vi "Folder Setting.vi"(8 "error in":errorcluster, 10 "Folder containing database files":path=path "C:/MHWirth/Data Logging Application/Logs/Database", 11 "Folder for saving log files":path=path "C:/MHWirth/Data Logging Application/Logs/Database") -> (0 "error out":errorcluster, 2 "database folder":path, 3 "TDMS folder":path)   [LabVIEW 2014]
doc: "<B>Copyrights</B>: (c) MHWirth 2015. All rights reserved.\n\nThis subVI updates the path for folders \"to save TDMS file\" and \"to contain the database\"."
panel:
  in  "update":bool
  # "Settings - Folder"
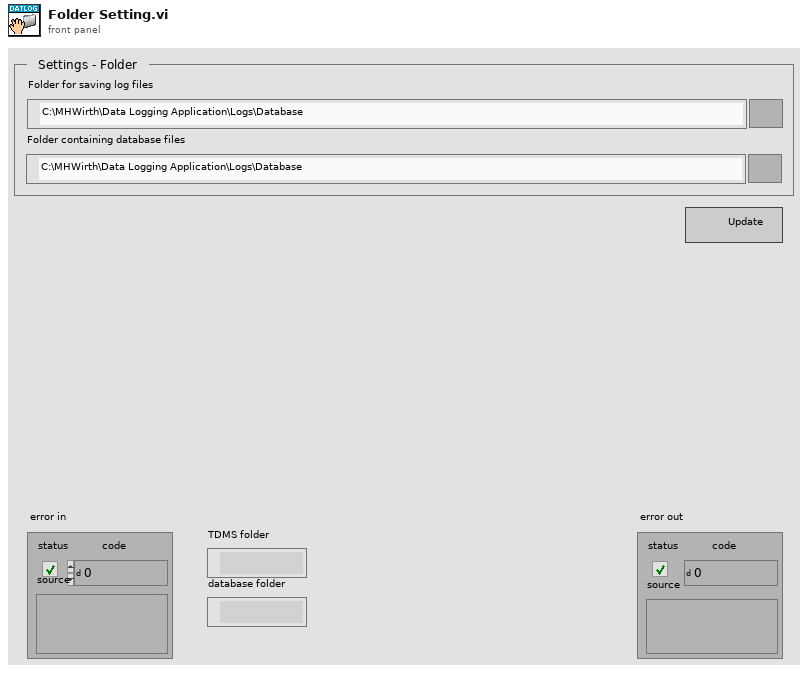
[diagram p1: front panel]
types:
  T1 = typedef "eventvkey.ctl" = enum16{"ASCII", "Enter", "Return", "Shift", "Ctrl", "Alt", "Cmd", "Opt", "Caps", "NumLock", "Clear", "Break", "Up", "Down", "Left", "Right", "Insert", "Delete", "Home", "End", "PageUp", "PageDown", "Escape", "Help", "Pause", "ScrollLock", "F1", "F2", "F3", "F4", "F5", "F6", "F7", "F8", "F9", "F10", "F11", "F12", "F13", "F14", "F15", "F16", "F17", "F18", "F19", "F20", "F21", "F22", "F23", "F24", "Play", "VolumeUp", "VolumeDown", "Mute", "Two Byte Char"}
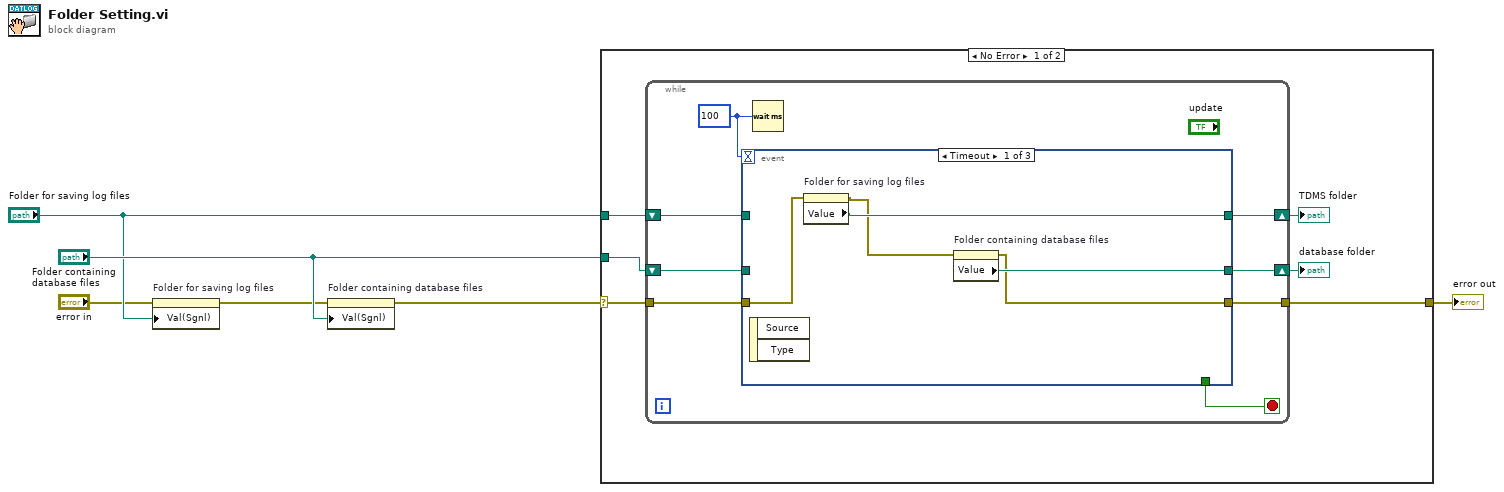
[diagram p0: block diagram]
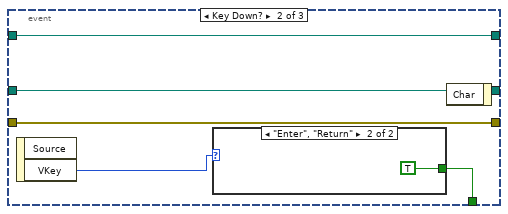
[diagram p2: hidden frame]
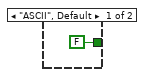
[diagram p3: hidden frame]
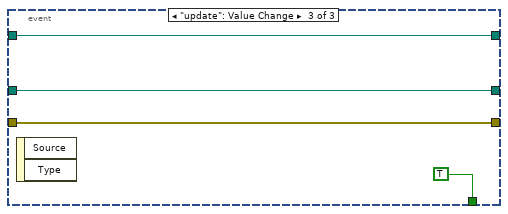
[diagram p4: hidden frame]
diagram:
  n1 = property on="Folder for saving log files" class="Path"(error in="error in", "Val(Sgnl)"="Folder for saving log files") -> (error out=w1:errorcluster)  [unwired: 1 in, 1 out]
  n2 = property on="Folder containing database files" class="Path"(error in=w1, "Val(Sgnl)"="Folder containing database files") -> (error out=w5:errorcluster)  [unwired: 1 in, 1 out]
  n3 = case shown="No Error" w5 {
    selector: w5 -> [w12 w37]
    tunnel: [w11 w37] -> w6
    tunnel: "Folder for saving log files" -> [w8 _]
    tunnel: "Folder containing database files" -> [w7 _]
    frame No Error {
      n4 = while {
        shift-right: [w17] -> w10
        shift-left: w8 -> [w20]
        shift-right: [w16] -> w9
        shift-left: w7 -> [w19]
        tunnel: w12 -> [w14]
        tunnel: [w13] -> w11
        stop <- w15 stop-if-true
        w18 = u32 100 ("milliseconds to wait")
        n5 = event shown="[0] Timeout" {
          selector: _ -> [_ _ _]
          dyn-events: _ -> [_ _ _]
          timeout: w18 -> [_ _ _]
          tunnel: w20 -> [_ w30 w34]
          tunnel: w19 -> [_ w29 w33]
          tunnel: [w23 w30 w34] -> w17
          tunnel: [w25 w29 w33] -> w16
          tunnel: [_ w27 TRUE] -> w15
          tunnel: w14 -> [w21 w28 w36]
          tunnel: [w24 w28 w36] -> w13
          event Timeout {
            n6 = event-data() -> ()  [unwired: 1 in, 2 out]
            n7 = property on="Folder for saving log files" class="Path"(error in=w21) -> (error out=w22:errorcluster, "Value"=w23:path)  [unwired: 1 in, 1 out]
            n8 = property on="Folder containing database files" class="Path"(error in=w22) -> (error out=w24:errorcluster, "Value"=w25:path)  [unwired: 1 in, 1 out]
          }
          event Key Down? {
            n9 = event-data() -> ("VKey"=w26:T1)  [unwired: 1 in, 1 out]
            n10 = case shown="\"Enter\", \"Return\"" w26 {
              tunnel: [FALSE TRUE] -> w27
              frame "ASCII", Default {
              }
              frame "Enter", "Return" {
              }
            }
            n11 = event-data() -> ()  [unwired: 2 in, 1 out]
          }
          event "update": Value Change {
            n12 = event-data() -> ()  [unwired: 1 in, 2 out]
          }
        }
        n13 = Wait (ms)(milliseconds to wait=w18) -> ()  [unwired: 1 out]
      }
      "TDMS folder" <- w10
      "database folder" <- w9
    }
    frame Error {
    }
  }
  "error out" <- w6
